vi "Pre Launch Init.vi"(11 "_Parent Actor Template in":refnum<class "_Parent Actor Template.lvclass">) -> (0 "error out":errorcluster, 3 "_Parent Actor Template out":refnum<class "_Parent Actor Template.lvclass">)   [LabVIEW 2016, in "_Parent Actor Template.lvlib" / "_Parent Actor Template.lvclass"]
doc: "(<B>Filename</B>: Actor Framework.lvlib:Actor.lvclass:Pre Launch Init.vi)\n\nDefines behavior that occurs after the Launch Actor method is invoked but before the actor's Actor Core method begins running.\n\nThe Pre Launch Init method is guaranteed to finish before the Launch Actor method returns to its caller and before the actor itself receives any messages. Any references that the Pre Launch Init method obtains are guaranteed to have the same lifetime as the actor itself. Any errors that the Pre Launch Init method returns will abort the launch.\n\nBy default, this method does nothing. A descendant class may override it to define behavior."
uses:
  _Parent Actor Template.lvclass
  <vilib>/ActorFramework/Actor/Actor.lvclass
  Enum - Debug Context.ctl
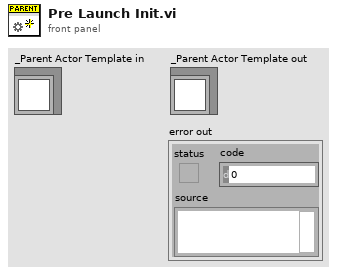
[diagram p1: front panel]
types:
  T1 = typedef "_Parent Actor Template.lvlib/_Parent Actor Template.lvclass/Enum - Debug Context.ctl" = enum16{"Null", "Startup", "Shutdown"}
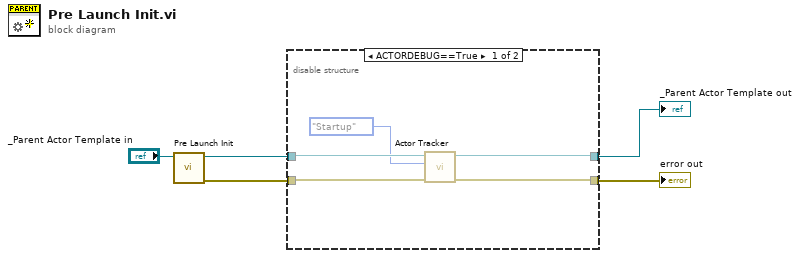
[diagram p0: block diagram]
diagram:
  n1 = call-parent "Pre Launch Init.vi"("Actor in"="_Parent Actor Template in") -> ("error out"=w5:errorcluster, "Actor out"=w2:refnum<class "_Parent Actor Template.lvclass">)  [unwired: 9 in]
  n2 = disable-structure shown="ACTORDEBUG==True" {
    disable-tunnel: w5 -> [w7 w12]
    disable-tunnel: [w8 w12] -> w3
    disable-tunnel: w2 -> [w9 w11]
    disable-tunnel: [w10 w11] -> w1
    frame condition #0 {
      n3 = call "Actor Tracker.vi"("error in"=w7, "Context"=Enum_-_Debug_Context."Startup", "_Parent Actor Template in"=w9) -> ("error out"=w8:errorcluster, "_Parent Actor Template out"=w10:refnum<class "_Parent Actor Template.lvclass">)  [unwired: 7 in]
    }
    frame condition #1 (active) {
    }
  }
  "error out" <- w3
  "_Parent Actor Template out" <- w1
